vi "Write Receiver Params.vi"(8 "error in (no error)":errorcluster, 9 "Image Receiver":refnum<class "Message Enqueuer.lvclass">, 10 "New Image Msg":refnum<class "New Image Msg.lvclass">, 11 "Camera in":refnum<class "Camera Actor.lvclass">) -> (0 "error out":errorcluster, 3 "Camera out":refnum<class "Camera Actor.lvclass">)   [LabVIEW 2020]
uses:
  Camera Actor.lvclass
  C:/Program Files (x86)/National Instruments/LabVIEW 2020/vi.lib/ActorFramework/Actor/Actor.lvclass
  C:/Users/AlexK/work/LabVIEW Programme/POLARIS-AS-3-Cams/Submodules/HIJ Vision/Camera Actors/Camera Actor/Camera Actor/Camera Actor.lvclass
  ICamera Messages/New Image Msg/New Image Msg.lvclass
  <vilib>/ActorFramework/Message Enqueuer/Message Enqueuer.lvclass
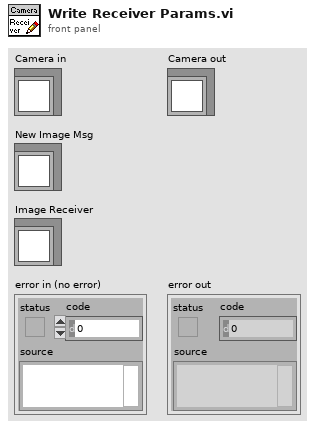
[diagram p1: front panel]
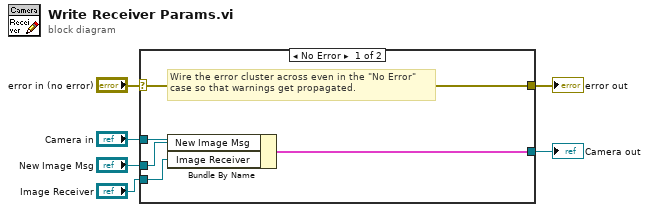
[diagram p0: block diagram]
diagram:
  n1 = case shown="No Error" "error in (no error)" {
    selector: "error in (no error)" -> [w10 w13]
    tunnel: [w10 w13] -> w5
    tunnel: [w9 w12] -> w3
    tunnel: "Camera in" -> [w11 w12]
    tunnel: "New Image Msg" -> [w8 _]
    tunnel: "Image Receiver" -> [w7 _]
    frame No Error {
      # "Wire the error cluster across even in the \"No Error\"\ncase so that warnings get propagated."
      n2 = Bundle By Name(cluster=w11, "New Image Msg"=w8, "Image Receiver"=w7) -> (w9:cluster{})
    }
    frame Error {
    }
  }
  "error out" <- w5
  "Camera out" <- w3
